vi "Find Sec Max.vi"(8 "Error Input":errorcluster, 11 "Input Array":i32[](array[numeric])=[6, 7, 8, 9]) -> (0 "Error Output":errorcluster, 2 "Second Largest":dbl, 3 "First Largest":dbl)   [LabVIEW 2024]
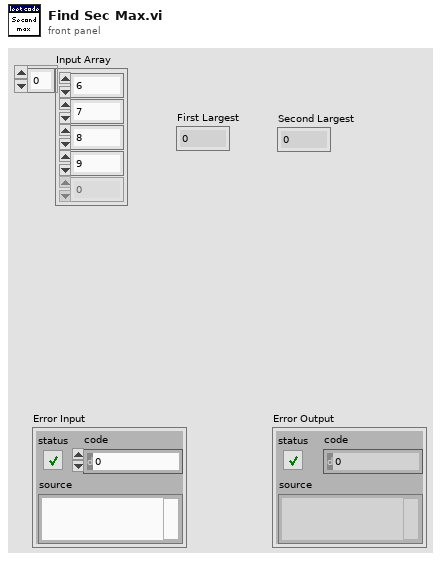
[diagram p1: front panel]
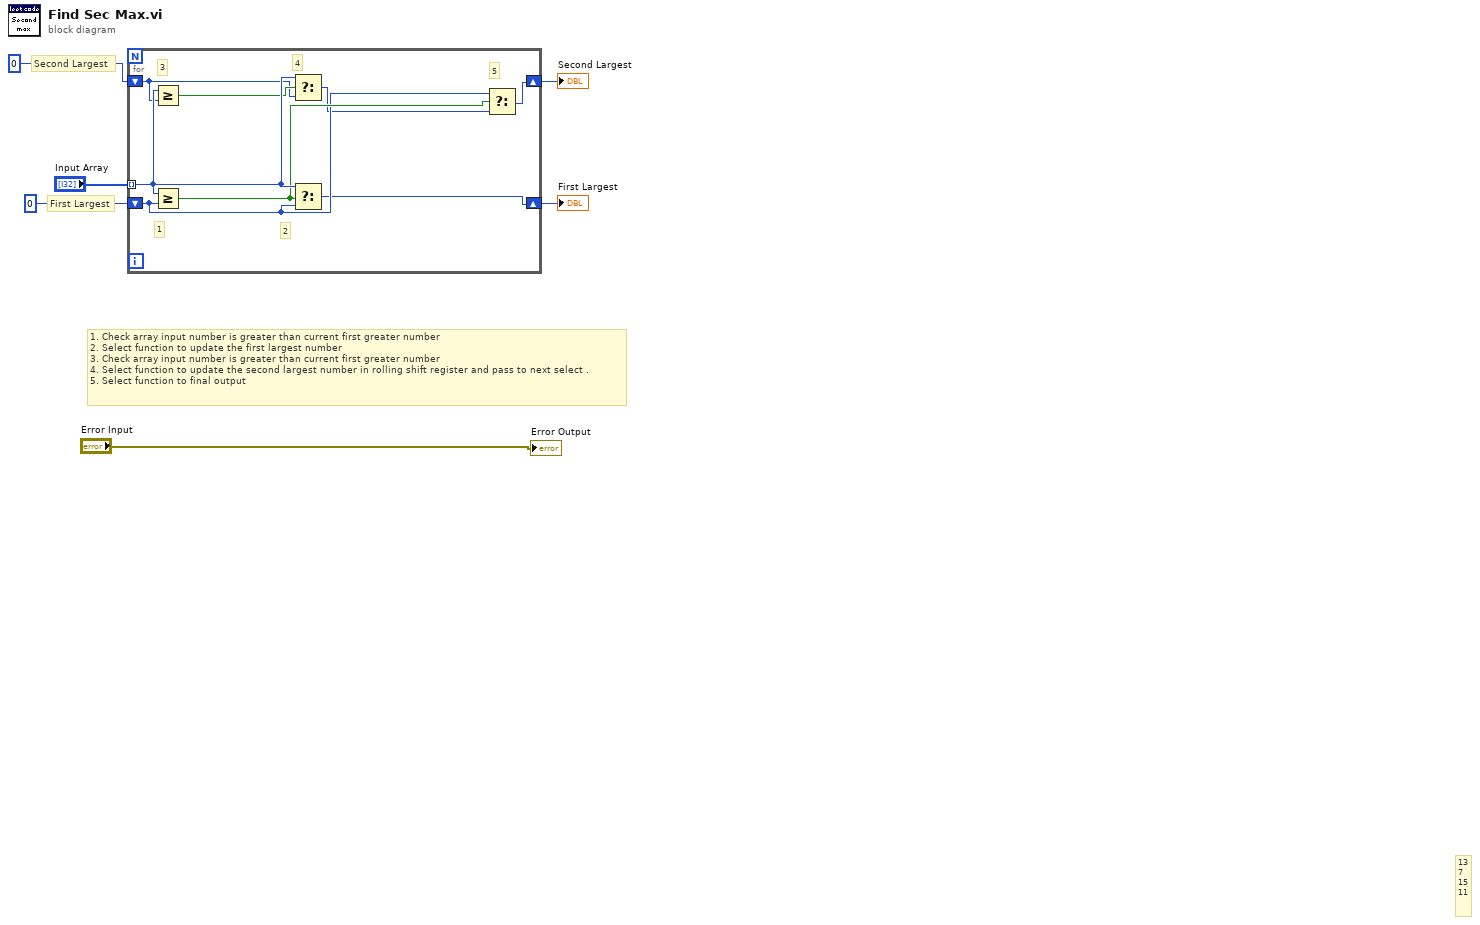
[diagram p0: block diagram]
diagram:
  # "1. Check array input number is greater than current first greater number \n2. Select function to update the first largest number \n3. Check array input number is greater than current first greater number\n4. Select function to update the second largest number in rolling shift register and pass to next select .\n5. Select function to final output"
  # "13\n7\n15\n11"
  # "Second Largest"
  # "First Largest"
  n1 = for {
    tunnel: "Input Array" -> [w14] mode=indexing
    shift-right: [w8] -> w3
    shift-left: 0 -> [w12]
    shift-right: [w7] -> w2
    shift-left: 0 -> [w10]
    # "5"
    # "4"
    # "3"
    # "2"
    # "1"
    n2 = Greater Or Equal?(x=w14, y=w12) -> (x >= y?=w13:bool)
    n3 = Greater Or Equal?(x=w14, y=w10) -> (x >= y?=w11:bool)
    n4 = Select(t=w14, s=w13, f=w12) -> (s? t:f=w9:i32)
    n5 = Select(t=w14, s=w11, f=w10) -> (s? t:f=w7:i32)
    n6 = Select(t=w10, s=w11, f=w9) -> (s? t:f=w8:i32)
  }
  "Second Largest" <- w3
  "First Largest" <- w2
  "Error Output" <- "Error Input"
